vi "Complex Lyapunov Equations.vi"(8 "equation type":i32(ring) items=["Continuous", "Discrete"], 9 "matrix type":i32(ring)=3 items=["General"=0, "Upper Triangular"=3], 10 "B":T1, 11 "A":T1) -> (0 "error":i32, 2 "scale":dbl=1.0, 3 "X":T1)   [LabVIEW 2017, in "NI_AALPro.lvlib"]
doc: "Solves the Lyapunov matrix equation. The data types you wire to the <B>A</B> and <B>B</B> inputs determine the polymorphic instance to use."
uses:
  <vilib>/Analysis/NI_AALPro.lvlib
  <vilib>/Analysis/Matrix/Datatypes/ComplexMatrix.ctl
  <resource>/lvanlys.dll
  <vilib>/Analysis/Matrix/NI_Matrix.lvlib
panel:
  # "Solve Lyapunov Equations"
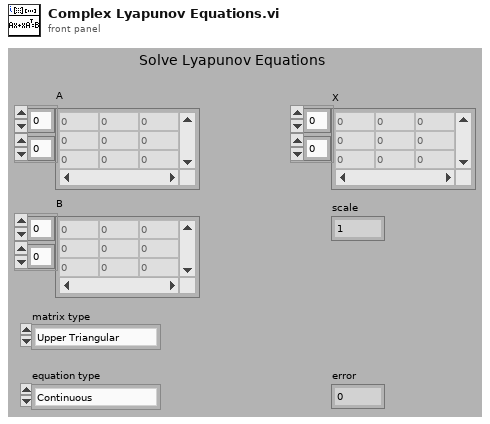
[diagram p1: front panel]
types:
  T1 = typedef "NI_Matrix.lvlib/ComplexMatrix.ctl" = cdb[][]
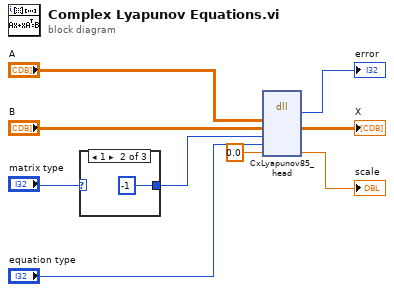
[diagram p0: block diagram]
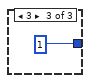
[diagram p3: hidden frame]
diagram:
  n1 = case shown="1" "matrix type" {
    selector: "matrix type" -> [w10 _ _]
    tunnel: [w10 -1 ("matrix type") 1] -> w4
    frame 0, Default {
    }
    frame 1 {
    }
    frame 3 {
    }
  }
  n2 = dll-call lib="e:/builds/penguin/labview/branches/2017/dev/dist/resource/lvanlys.*" fn="CxLyapunov85_head"("aH"="A", "bH"="B", "type"=w4, "eqtype"="equation type", "scale"=0.0) -> ("return type"=→"error":i32, "bH"=→"X":T1, "scale"=→"scale":dbl)  [unwired: 6 in, 2 out]
